vi "GetCtlValue_Core.vi"(8 "error in (no error)":errorcluster, 10 "CtlName In":string, 11 "ctlRef_Maps in":refnum<class "ctlRef_Maps.lvclass">) -> (0 "error out":errorcluster, 1 "Value":variant, 3 "ctlRef_Maps out":refnum<class "ctlRef_Maps.lvclass">)   [LabVIEW 2020, in "CtlReferences.lvlib" / "ctlRef_Maps.lvclass"]
uses:
  ctlRef_Maps.lvclass
  C:/Viviota/Projects/VIV_ctlReferences/CtlReferences/CtlReferences.lvclass
  ctlRef_Maps.lvclass/ctlRef_Maps.ctl
  CtlReferences/CtlReferences.lvclass/CtlReferences.ctl
  CtlReferences/Read VIRef.vi
  CtlReferences/CtlReferences.lvclass
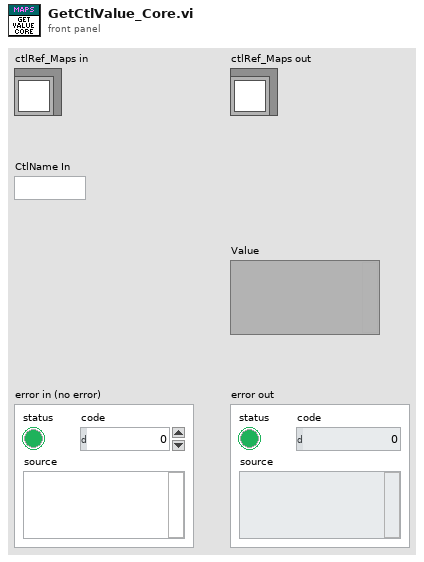
[diagram p1: front panel]
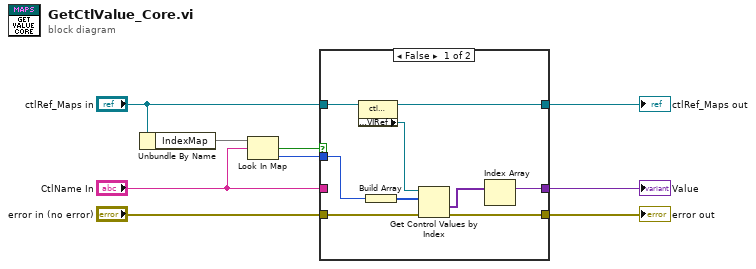
[diagram p0: block diagram]
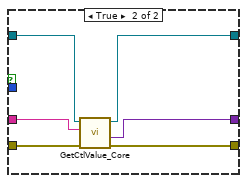
[diagram p2: hidden frame]
diagram:
  n1 = Unbundle By Name("ctlRef_Maps in") -> ("IndexMap"=w4:map{string, i32})
  n2 = Look In Map(map=w4, key="CtlName In") -> (key not found?=w2:bool, value=w1:i32)  [unwired: 1 in]
  n3 = case shown="False" w2 {
    tunnel: [w16 w24] -> w9
    tunnel: [w10 w23] -> w8
    tunnel: [w13 w22] -> w7
    tunnel: "error in (no error)" -> [w17 w21]
    tunnel: "ctlRef_Maps in" -> [w18 w20]
    tunnel: "CtlName In" -> [_ w19]
    tunnel: w1 -> [w15 _]
    frame False {
      n4 = property class="ctlRef_Maps.lvclass"(reference=w18) -> (reference out=w13:refnum<class "ctlRef_Maps.lvclass">, "Accessors:VIRef"=w12:refnum<vi>)  [unwired: 1 in, 1 out]
      n5 = Build Array(w15) -> (w14:i32[])
      n6 = Get Control Values by Index(0:w12, 1:w14, 3:w17) -> (10:w11:variant[], 11:w16:errorcluster)
      n7 = Index Array(array=w11) -> (element=w10:variant)  [unwired: 1 in]
    }
    frame True {
      n8 = call-parent "GetCtlValue_Core.vi"("error in (no error)"=w21, "CtlName In"=w19, "CtlReferences in"=w20) -> ("error out"=w24:errorcluster, "Value"=w23:variant, "CtlReferences out"=w22:refnum<class "ctlRef_Maps.lvclass">)  [unwired: 6 in]
    }
  }
  "ctlRef_Maps out" <- w7
  "error out" <- w9
  "Value" <- w8
